vi "Write Element of Term.vi"(8 "error in (no error)":errorcluster, 9 "Termination":refnum<class "Termination.lvclass">, 10 "index":i32, 11 "State in":refnum<class "State.lvclass">) -> (0 "error out":errorcluster, 3 "State out":refnum<class "State.lvclass">)   [LabVIEW 2020, in "State.lvclass"]
uses:
  State.lvclass
  Termination/Termination.lvclass
  State.lvclass/State.ctl
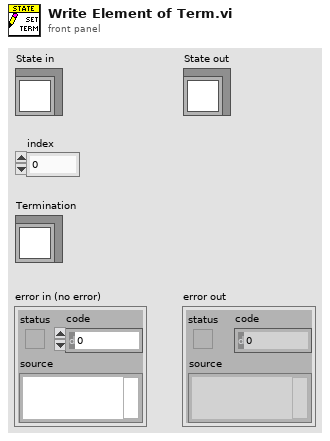
[diagram p1: front panel]
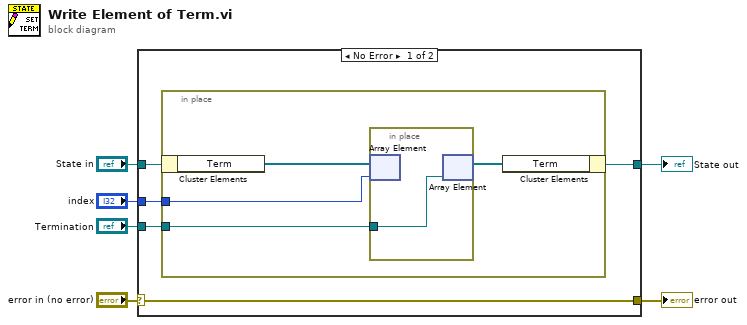
[diagram p0: block diagram]
diagram:
  n1 = case shown="No Error" "error in (no error)" {
    selector: "error in (no error)" -> [w11 w17]
    tunnel: [w11 w17] -> w5
    tunnel: [w9 w18] -> w3
    tunnel: "State in" -> [w7 w18]
    tunnel: "Termination" -> [w8 _]
    tunnel: "index" -> [w10 _]
    frame No Error {
      n2 = in-place {
        in-place-border: w10 -> [w14]
        in-place-border: w8 -> [w12]
        n3 = in-place-cluster #1(w7) -> ("Term"=w15:refnum<class "Termination.lvclass">[])
        n4 = in-place {
          in-place-border: w12 -> [w16]
          n5 = in-place-array #2(w15, w14) -> ()  [unwired: 1 out]
          n6 = in-place-array #2(w16) -> (w13:refnum<class "Termination.lvclass">[])  [unwired: 1 out]
        }
        n7 = in-place-cluster #1("Term"=w13) -> (w9:refnum<class "State.lvclass">)
      }
    }
    frame Error {
    }
  }
  "error out" <- w5
  "State out" <- w3
